vi "Get Port Incoming Section.vi"(8 "error in":errorcluster, 11 "ports ref":T1 format="%.0x") -> (0 "error out":errorcluster, 2 "incoming ref out":T1 format="%.0x", 3 "ports ref out":T1 format="%.0x", 4 "found?":bool)   [LabVIEW 2020, in "AIM ARINC 664 Scripting.lvlib"]
uses:
  AIM ARINC 664 Scripting.lvlib
  <vilib>/NI VeriStand/Custom Device API/Custom Device Item Ref.ctl
  Constants.vi
  <vilib>/NI VeriStand/Custom Device Tools/Custom Device Utility Library/NI VeriStand - Search for Item by GUID.vi
  <vilib>/NI VeriStand/Custom Device Tools/Custom Device Utility Library/Custom Device Utility Library.lvlib
  <vilib>/NI VeriStand/Custom Device API/Custom Device API.lvlib
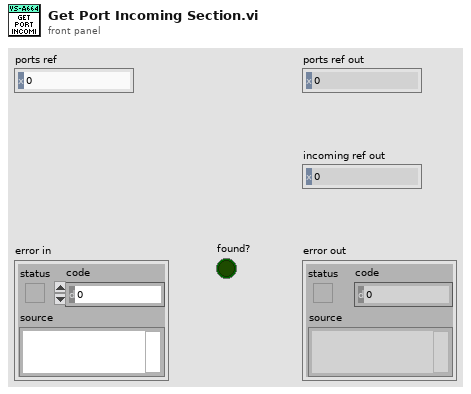
[diagram p1: front panel]
types:
  T1 = typedef "Custom Device API.lvlib/Custom Device Item Ref.ctl" = u64
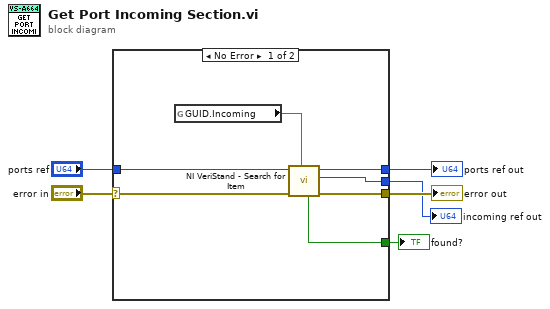
[diagram p0: block diagram]
diagram:
  n1 = case shown="No Error" "error in" {
    selector: "error in" -> [w11 w15]
    tunnel: "ports ref" -> [w13 w14]
    tunnel: [w10 w15] -> w5
    tunnel: [w9 w14] -> w4
    tunnel: [w8 _] -> w2
    tunnel: [w7 _] -> w1
    frame No Error {
      n2 = global read "Constants.vi" "GUID.Incoming"() -> (w12:string)
      n3 = call-poly <vilib>:"NI VeriStand - Search for Item.vi"("error in"=w11, "Item GUID"=w12, "Section Ref in"=w13) -> ("error out"=w10:errorcluster, "Item Ref"=w8:T1, "Section Ref out"=w9:T1, "Found"=w7:bool)  [unwired: 5 in]
    }
    frame Error {
    }
  }
  "error out" <- w5
  "ports ref out" <- w4
  "incoming ref out" <- w2
  "found?" <- w1
